vi "Shooter Controller.vi"(8 "error in":errorcluster) -> ()   [LabVIEW 2020]
doc: "This VI executes continuously carrying out the current operation and responding to updates or new operations. It will often contain the timing or control code that is difficult to place directly in TeleOp. This VI generally opens all sensors and motors and isolates the rest of the robot code from knowing how the operations are carried out."
uses:
  <vilib>/Rock Robotics/WPI/Framework/Completion Status.ctl
  Shooter Setpoints.ctl
  Shooter Operations.ctl
  <vilib>/Rock Robotics/WPI/ThirdParty/Phoenix-LabVIEW/Motor Controller/Controls/CTRE_Phoenix_MotorControl_ControlMode.ctl
  <vilib>/Rock Robotics/WPI/ThirdParty/Phoenix-LabVIEW/Motor Controller/Get/CTRE_Phoenix_MotorController_GetSelectedSensorData.vi
  vi's/Global Variables.vi
  <vilib>/Rock Robotics/Network Tables/NT Write Boolean.vi
panel:
  in  "Interactive Values":T1 {"Control Mode" items=["PercentOutput"=0, "Position"=1, "Velocity"=2, "Current"=3, "Follower"=5, "MotionProfile"=6, "MotionMagic"=7, "MotionProfileArc"=10, "Disabled"=15]}
  out "Current\nCmd":string
  in  "Buttons":cluster{"Execute Cmd":bool, "Abort Cmd":bool}
  out "Command Timing":cluster{"Start Time (ms)":u32, "Iterations":i32}
  out "Status":T4
  # "Tip: It may be helpful to observe inputs and sensor values.\nYou may also want to display tuning or debugging controls."
  # "Interactive Command: You may fill in the settings for a command\nand schedule it with the Execute button. You can observe and abort\nany command while fine tuning the code for the controller."
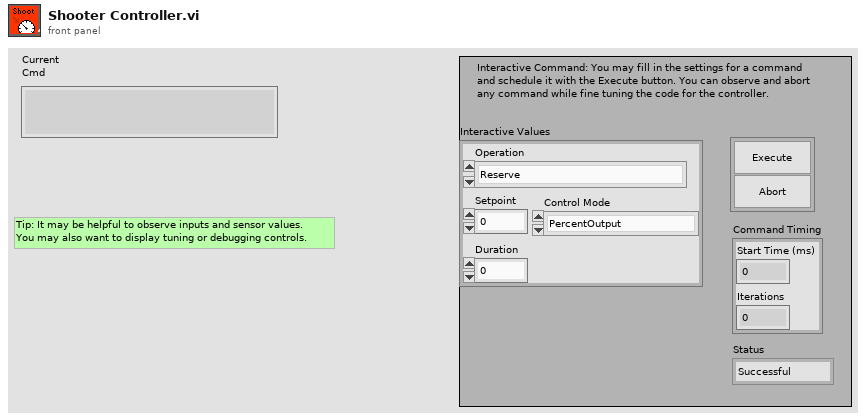
[diagram p1: front panel]
types:
  T1 = typedef "Shooter Setpoints.ctl" = cluster{"Operation":T2, "Setpoint":dbl, "Duration":dbl, "Control Mode":T3}
  T2 = typedef "Shooter Operations.ctl" = enum16{"Reserve", "Read Current", "Immediate"}
  T3 = typedef "CTRE_Phoenix_MotorControl_ControlMode.ctl" = u16
  T4 = typedef "Completion Status.ctl" = enum16{"Successful", "Aborted", "Incomplete"}
  T5 = typedef "WPI_MotorControlDeviceRef.ctl" = cluster{"DeviceStatus":errorcluster, "Type":T6, "PWM":cluster{"PWM Channel":T7, "DeadBand":T8}, "CAN":cluster{"Device Number":u8, "SetOutput VI Ref":variant, "GetOutput VI Ref":variant, "Enable VI Ref":variant, "Disable VI Ref":variant, "Data":variant}, "Invert":bool, "DIO PWM":cluster{"PWM \"Enable\" Channel":T7, "DIOChannel":T9, "PWM Rate":dbl}}
  T6 = typedef "WPI_MotorControlType.ctl" = enum16{"PWM", "CAN", "DIO PWM"}
  T7 = typedef "FPGA_DIOPWMChannel.ctl" = enum8{"PWM 0", "PWM 1", "PWM 2", "PWM 3", "PWM 4", "PWM 5", "PWM 6", "PWM 7", "PWM 8", "PWM 9", "PWM MXP 0", "PWM MXP 1", "PWM MXP 2", "PWM MXP 3", "PWM MXP 4", "PWM MXP 5", "PWM MXP 6", "PWM MXP 7", "PWM MXP 8", "PWM MXP 9", "Invalid"}
  T8 = typedef "WPI_PWMDeadband.ctl" = cluster{"Name":string, "maxPositivePwm":i32, "minPositivePwm":i32, "centerPwm":i32, "maxNegativePwm":i32, "minNegativePwm":i32, "angularRange":u16}
  T9 = typedef "FPGA_DIOChannel.ctl" = enum8{"DIO 0", "DIO 1", "DIO 2", "DIO 3", "DIO 4", "DIO 5", "DIO 6", "DIO 7", "DIO 8", "DIO 9", "DIO MXP 0", "DIO MXP 1", "DIO MXP 2", "DIO MXP 3", "DIO MXP 4", "DIO MXP 5", "DIO MXP 6", "DIO MXP 7", "DIO MXP 8", "DIO MXP 9", "DIO MXP 10", "DIO MXP 11", "DIO MXP 12", "DIO MXP 13", "DIO MXP 14", "DIO MXP 15", "SPI Port CS1", "SPI Port CS2", "SPI Port CS3", "SPI Port MISO", "SPI Port MOSI", "Invalid"}
  T10 = typedef "Command Status Info.ctl" = cluster{"Name":string, "Status":T4, "notifier out":T11}
  T11 = typedef "Completion Notifier.ctl" = refnum<notifier>
  T12 = cluster{"Current Command":T1, "Command Timing":cluster{"Start Time (ms)":u32, "Iterations":i32}, "Command Arguments":cluster{"Command Info":T10, "Description":string, "Default Command":T1, "queue out":refnum<queue>, "Subsystem Name":string}}
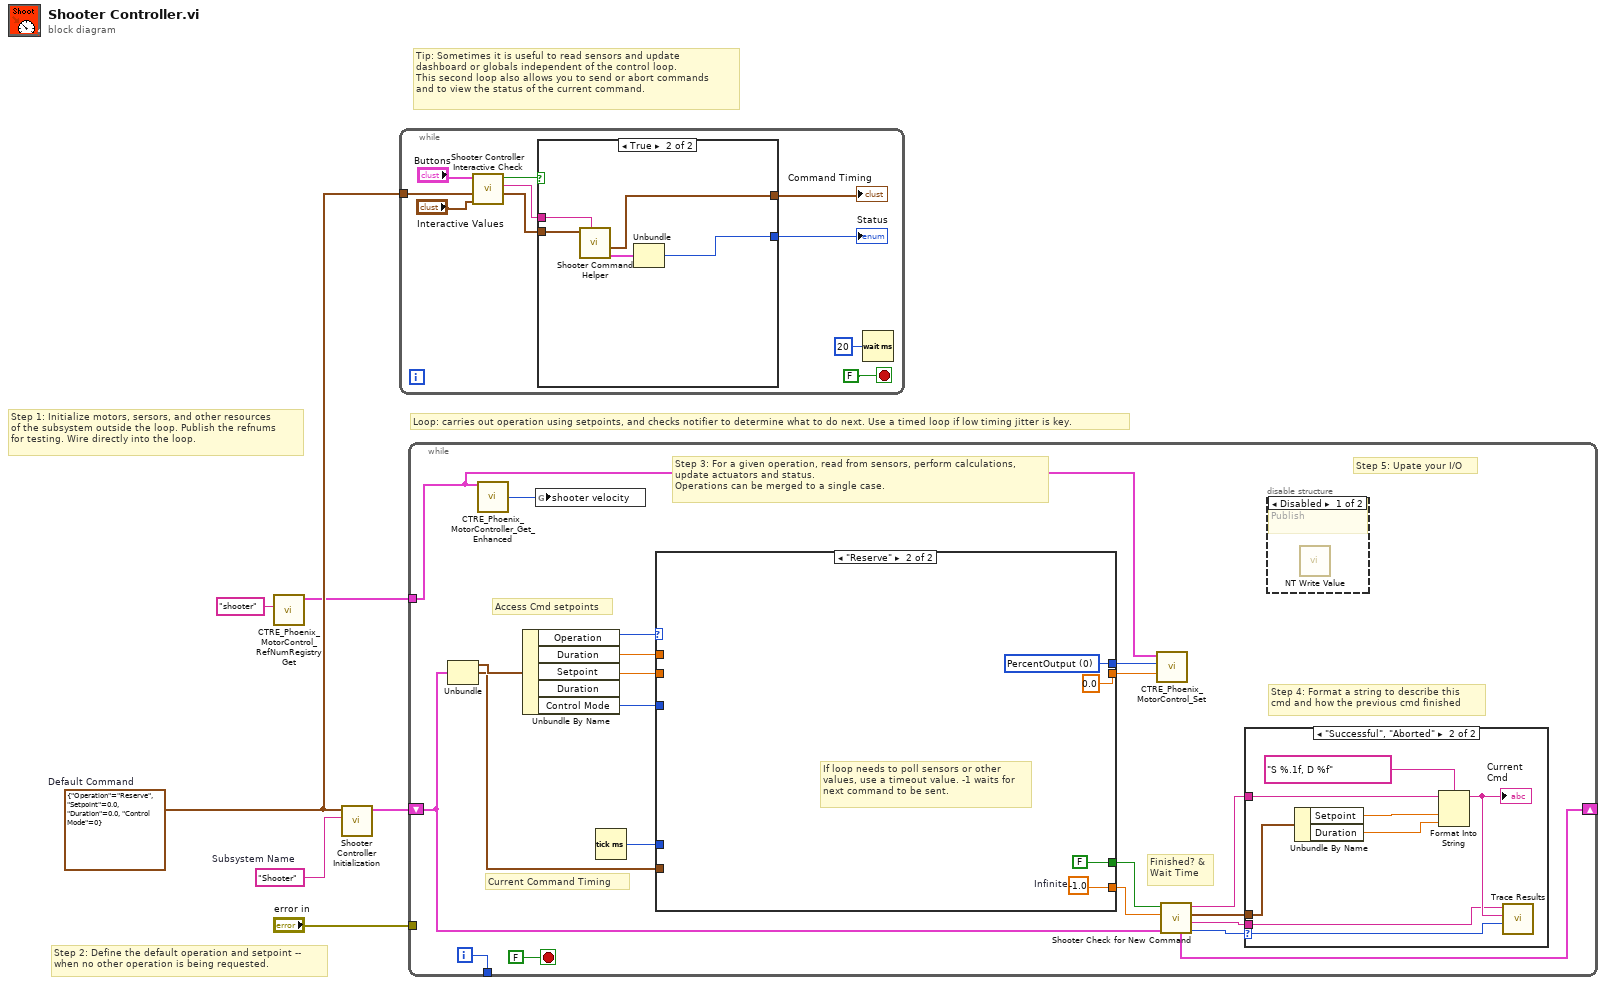
[diagram p0: block diagram]
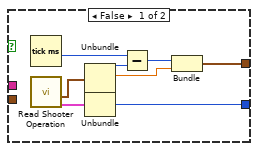
[diagram p2: hidden frame]
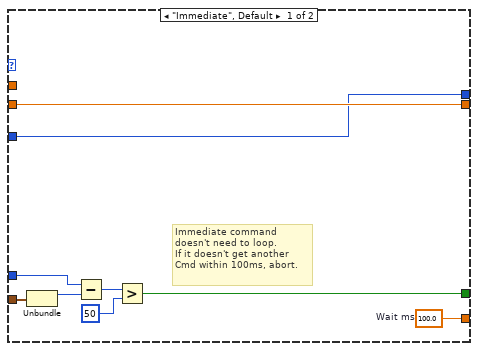
[diagram p5: hidden frame]
diagram:
  w3 = T1 {"Operation"=enum."Reserve", "Setpoint"=0.0, "Duration"=0.0, "Control Mode"=0}  # Default Command
  w4 = "Shooter"  # Subsystem Name
  # "Tip: Sometimes it is useful to read sensors and update\ndashboard or globals independent of the control loop.\nThis second loop also allows you to send or abort commands\nand to view the status of the current command."
  # "Step 2: Define the default operation and setpoint --\nwhen no other operation is being requested."
  # "Step 1: Initialize motors, sersors, and other resources\nof the subsystem outside the loop. Publish the refnums\nfor testing. Wire directly into the loop."
  # "Loop: carries out operation using setpoints, and checks notifier to determine what to do next. Use a timed loop if low timing jitter is key."
  n1 = call <vilib>:"CTRE_Phoenix_MotorControl_RefNumRegistryGet.vi"("refnum name"="shooter") -> ("PhoenixMotorControlDevRef"=w1:T5)  [unwired: 9 in, 1 out]
  n2 = call "Shooter Controller Initialization.vi"("Subsystem Name"=w4, "Default Command"=w3) -> ("Current Command"=w5:T12)  [unwired: 9 in]
  n3 = while {
    tunnel: w3 -> [w13]
    stop <- FALSE stop-if-true
    n4 = call "Shooter Controller Interactive Check.vi"("Interactive Command in"="Interactive Values", "Default Command"=w13, "Buttons"="Buttons") -> ("Interactive Command out"=w10:T1, "Trace String"=w11:string, "Schedule"=w12:bool)  [unwired: 6 in]
    n5 = case shown="True" w12 {
      tunnel: [w24 w29] -> w9
      tunnel: w10 -> [_ w27]
      tunnel: [w20 w25] -> w8
      tunnel: w11 -> [_ w28]
      frame False {
        n6 = Tick Count (ms)() -> (millisecond timer value=w19:u32)
        n7 = call "Read Shooter Operation.vi"() -> ("Command Info"=w17:T10, "SubSystem Data"=w18:T1)  [unwired: 9 in, 1 out]
        n8 = Unbundle(w18) -> ("Operation"=w23:T2, "Setpoint"=w21:dbl)  [unwired: 2 out]
        n9 = Unbundle(w17) -> ("Status"=w24:T4)  [unwired: 2 out]
        n10 = Subtract(x=w19, y=w23) -> (x-y=w22:u32)
        n11 = Bundle(w22, "Setpoint"=w21) -> (w20:cluster{u32, "Setpoint":dbl})  [unwired: 1 in]
      }
      frame True {
        n12 = call "Shooter Command Helper.vi"("Description"=w28, "SubSystem Data"=w27) -> ("Command Info Out"=w26:T10, "Command Timing"=w25:cluster{"Start Time (ms)":u32, "Iterations":i32})  [unwired: 7 in, 1 out]
        n13 = Unbundle(w26) -> ("Status"=w29:T4)  [unwired: 2 out]
      }
    }
    "Status" <- w9
    "Command Timing" <- w8
    n14 = Wait (ms)(milliseconds to wait=u32 20) -> ()  [unwired: 1 out]
  }
  n15 = while {
    shift-right: [w42] -> _
    shift-left: w5 -> [w35]
    tunnel: [w49] -> _
    tunnel: "error in" -> [_]
    tunnel: w1 -> [w30]
    i -> [w49]
    stop <- FALSE stop-if-true
    # "Step 5: Upate your I/O"
    # "Step 4: Format a string to describe this\ncmd and how the previous cmd finished"
    # "Current Command Timing"
    # "Access Cmd setpoints"
    # "Finished? &\nWait Time"
    # "Step 3: For a given operation, read from sensors, perform calculations,\nupdate actuators and status.\nOperations can be merged to a single case."
    n16 = Unbundle(w35) -> ("Current Command"=w48:T1, "Command Timing"=w44:cluster{"Start Time (ms)":u32, "Iterations":i32})  [unwired: 1 out]
    n17 = call-poly <vilib>:"CTRE_Phoenix_MotorController_Get_Enhanced.vi"("PhoenixMotorControlDevRef"=w30) -> ("Velocity (Raw Sensor Units per 100 ms)"=w34:i32)  [unwired: 11 in, 3 out]
    n18 = Unbundle By Name(w48) -> ("Operation"=w47:T2, "Duration"=w46:dbl, "Setpoint"=w43:dbl, "Control Mode"=w32:T3)  [unwired: 1 out]
    n19 = global write "Global Variables.vi" "shooter velocity"(w34) -> ()
    n20 = Tick Count (ms)() -> (millisecond timer value=w45:u32)
    n21 = case shown="\"Reserve\"" w47 {
      tunnel: [w67 w71] -> w40
      tunnel: [w61 FALSE ("ignore previous (F)")] -> w41
      tunnel: w44 -> [w63 _]
      tunnel: w46 -> [_ _]
      tunnel: w45 -> [w62 _]
      tunnel: w43 -> [w60 _]
      tunnel: [w60 0.0 ("Setpoint")] -> w33
      tunnel: w32 -> [w59 _]
      tunnel: [w59 w69] -> w31
      frame "Immediate", Default {
        w67 = 100.0  # Wait ms
        # "Immediate command\ndoesn't need to loop.\nIf it doesn't get another\nCmd within 100ms, abort."
        n22 = Unbundle(w63) -> ("Start Time (ms)"=w66:u32)  [unwired: 1 out]
        n23 = Subtract(x=w62, y=w66) -> (x-y=w65:u32)
        n24 = Greater?(x=w65, y=u8 50 ("Left Motor")) -> (0:w61:bool)
      }
      frame "Reserve" {
        w69 = T3 0 items=["PercentOutput"=0, "Position"=1, "Velocity"=2, "Current"=3, "Follower"=5, "MotionProfile"=6, "MotionMagic"=7, "MotionProfileArc"=10, "Disabled"=15] ("Control Mode")
        w71 = -1.0  # Infinite
        # "If loop needs to poll sensors or other\nvalues, use a timeout value. -1 waits for\nnext command to be sent."
      }
    }
    n25 = call <vilib>:"CTRE_Phoenix_MotorControl_Set.vi"("Output"=w33, "Control Mode"=w31, "PhoenixMotorControlDevRef"=w30) -> ()  [unwired: 7 in, 2 out]
    n26 = call "Shooter Check for New Command.vi"("Current Command"=w35, "Wait time (ms)"=w40, "Finished?"=w41) -> ("Completion"=w36:T4, "Subsystem Name"=w37:string, "Current Command"=w38:T1, "Initial Trace String"=w39:string, "NextCommand"=w42:T12)  [unwired: 4 in]
    n27 = case shown="\"Successful\", \"Aborted\"" w36 {
      selector: w36 -> [_ w58]
      tunnel: w39 -> [_ w54]
      tunnel: w38 -> [_ w55]
      tunnel: w37 -> [_ w51]
      frame "Incomplete", Default {
        # "Continuing current command"
      }
      frame "Successful", "Aborted" {
        # "Report and setup for next command"
        n28 = Unbundle By Name(w55) -> ("Setpoint"=w57:dbl, "Duration"=w52:dbl)
        n29 = Format Into String(format string="S %.1f, D %f", initial string=w54, w57, w52) -> (resulting string=w53:string)  [unwired: 1 in, 1 out]
        "Current\nCmd" <- w53
        n30 = call <vilib>:"Trace Results.vi"("Status of previous command"=w58, "Description"=w53, "Subsystem"=w51) -> ()  [unwired: 9 in]
      }
    }
    n31 = disable-structure shown="Disabled" {
      frame Disabled {
        # "Publish"
        n32 = call-poly <vilib>:"NT Write Value.vi"() -> ()  [unwired: 11 in, 1 out]
      }
      frame Enabled {
      }
    }
  }
